vi "Math-Truncated Exponential RNG.vi"(0 "samples":i32, 5 "Min":dbl, 7 "Max":dbl, 9 "Lambda":dbl, 12 "seed":i32=-1) -> (4 "Array":dbl[](array[numeric]))   [LabVIEW 2020]
uses:
  <vilib>/gmath/statdist.llb/Uniform Random.vi
  <vilib>/gmath/NI_Gmath.lvlib
  <vilib>/Analysis/NI_AALBase.lvlib
panel:
  out "Histogram":T1(graph)
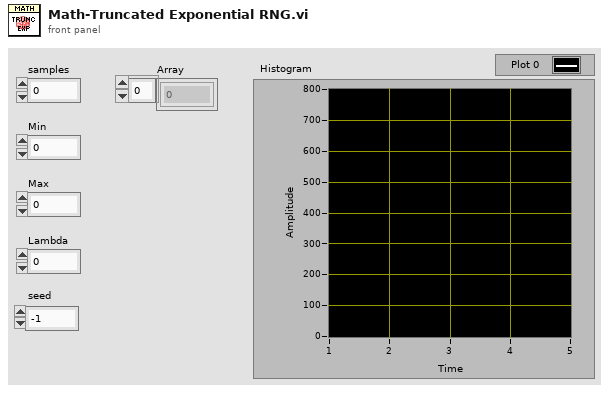
[diagram p1: front panel]
types:
  T1 = cluster{"X Values":dbl[], "Histogram: h(x)":i32[]}
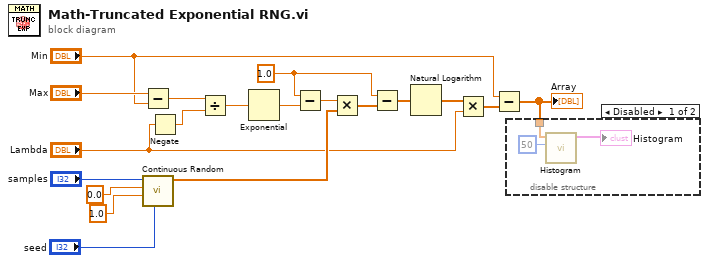
[diagram p0: block diagram]
diagram:
  w8 = 1.0
  n1 = Subtract(x="Max", y="Min") -> (x-y=w15:dbl)
  n2 = call-poly <vilib>:"Continuous Random.vi"("seed"="seed", "xmax"=1.0, "xmin"=0.0, "samples"="samples") -> ("uniform random data"=w10:dbl[])  [unwired: 6 in, 1 out]
  n3 = Negate(x="Lambda") -> (-x=w14:dbl)
  n4 = Divide(x=w15, y=w14) -> (x/y=w13:dbl)
  n5 = Exponential(1:w13) -> (0:w12:dbl)
  n6 = Subtract(x=w8, y=w12) -> (x-y=w11:dbl)
  n7 = Multiply(x=w11, y=w10) -> (x*y=w9:dbl[])
  n8 = Subtract(x=w8, y=w9) -> (x-y=w7:dbl[])
  n9 = Natural Logarithm(1:w7) -> (0:w6:dbl[])
  n10 = Multiply(x=w6, y="Lambda") -> (x*y=w4:dbl[])
  n11 = Subtract(x="Min", y=w4) -> (x-y=w2:dbl[])
  "Array" <- w2
  n12 = disable-structure shown="Disabled" {
    disable-tunnel: w2 -> [w22 _]
    frame Disabled {
      n13 = call <vilib>:"Histogram.vi"("intervals"=50, "X"=w22) -> ("Histogram Graph"=→"Histogram":T1)  [unwired: 6 in, 3 out]
    }
    frame Enabled {
    }
  }
